vi "sort_by.vi"(10 "column index":i32, 11 "data IN":dbl[][](array[numeric])) -> (3 "data OUT":dbl[][](array[numeric]))   [LabVIEW 2017, in "tools.lvlib"]
uses:
  tools.lvlib
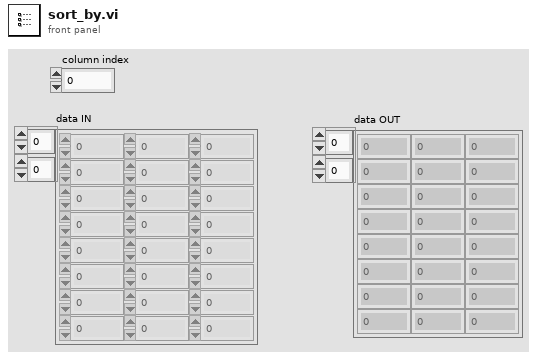
[diagram p1: front panel]
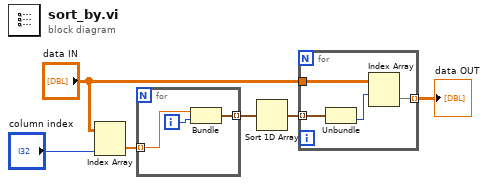
[diagram p0: block diagram]
diagram:
  n1 = Index Array(array="data IN", index (col)="column index") -> (element=w3:dbl[])  [unwired: 1 in]
  n2 = for {
    tunnel: w3 -> [w7] mode=indexing
    tunnel: [w8] -> w6 mode=indexing
    i -> [w9]
    n3 = Bundle("Numeric"=w7, w9) -> (w8:cluster{"Numeric":dbl, i32})  [unwired: 1 in]
  }
  n4 = Sort 1D Array(array=w6) -> (sorted array=w5:cluster{"Numeric":dbl, i32}[])
  n5 = for {
    tunnel: w5 -> [w13] mode=indexing
    tunnel: [w11] -> w1 mode=indexing
    tunnel: "data IN" -> [w10]
    n6 = Unbundle(w13) -> (w12:i32)  [unwired: 1 out]
    n7 = Index Array(array=w10, index (row)=w12) -> (element=w11:dbl[])  [unwired: 1 in]
  }
  "data OUT" <- w1
